vi "WaitForConnect.vi"(8 "error in (no error)":errorcluster, 11 "ServiceManager-Comms in":refnum<class "ServiceManager-Comms.lvclass">) -> (0 "error out":errorcluster, 3 "ServiceManager-Comms out":refnum<class "ServiceManager-Comms.lvclass">)   [LabVIEW 2020, in "ServiceManager.lvlib" / "ServiceManager-Comms.lvclass"]
uses:
  ServiceManager-Comms.lvclass
  C:/Program Files (x86)/National Instruments/LabVIEW 2020/vi.lib/ActorFramework/Actor/Actor.lvclass
  ServiceManager-Comms.lvclass/ServiceManager-Comms.ctl
  ServiceManager-Comms Messages/WaitForCommand Msg/WaitForCommand Msg.lvclass
  C:/Program Files (x86)/National Instruments/LabVIEW 2020/vi.lib/ActorFramework/Message/Message.lvclass
  ServiceManager-Comms Messages/WaitForConnect Msg/WaitForConnect Msg.lvclass
  <vilib>/ActorFramework/Actor/Actor.lvclass/Actor.ctl
  <vilib>/ActorFramework/Message Enqueuer/Message Enqueuer.lvclass/Message Enqueuer.ctl
  <vilib>/ActorFramework/Message Enqueuer/Init from Existing Queue.vi
  <vilib>/ActorFramework/Message Enqueuer/Message Enqueuer.lvclass
  <vilib>/ActorFramework/Actor/Actor.lvclass
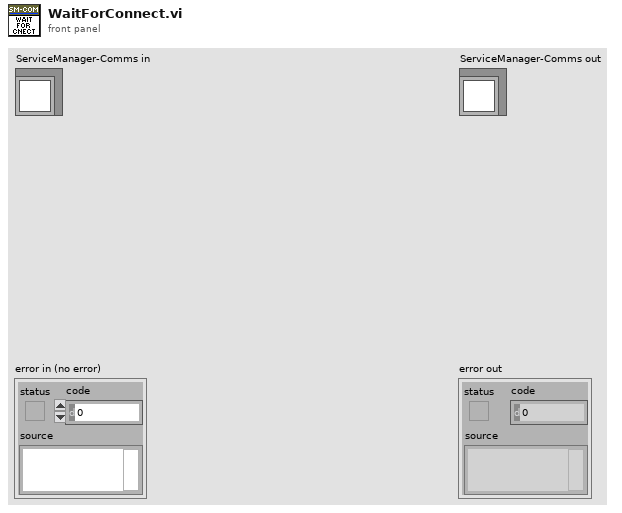
[diagram p1: front panel]
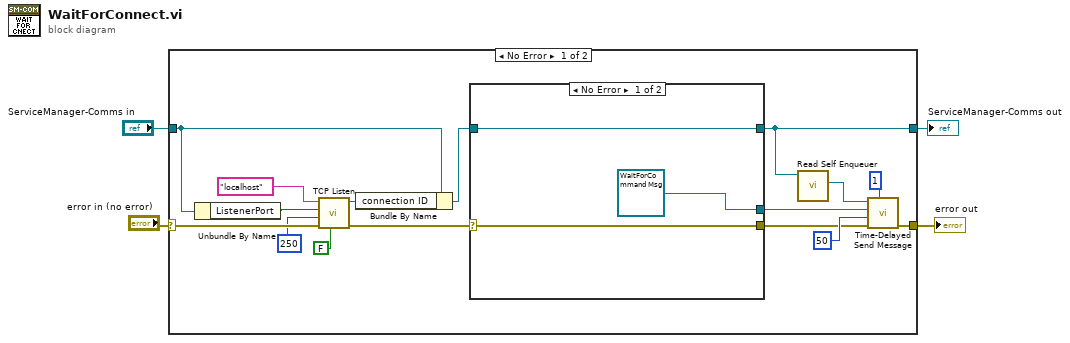
[diagram p0: block diagram]
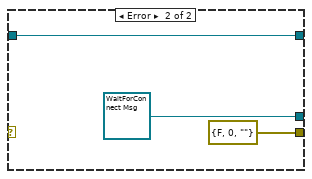
[diagram p2: hidden frame]
diagram:
  n1 = case shown="No Error" "error in (no error)" {
    selector: "error in (no error)" -> [w19 w28]
    tunnel: [w10 w28] -> w3
    tunnel: [w11 w27] -> w1
    tunnel: "ServiceManager-Comms in" -> [w16 w27]
    frame No Error {
      n2 = Unbundle By Name(w16) -> ("ListenerPort"=w18:u16)
      n3 = call <vilib>:"TCP Listen.vi"("resolve remote address (T)"=FALSE, "error in (no error)"=w19, "timeout ms (wait forever: -1)"=250, "port"=w18, "service name"="localhost") -> ("error out"=w13:errorcluster, "connection ID"=w15:refnum<k5>)  [unwired: 2 in, 3 out]
      n4 = Bundle By Name(cluster=w16, "connection ID"=w15) -> (w12:refnum<class "ServiceManager-Comms.lvclass">)
      n5 = case shown="No Error" w13 {
        selector: w13 -> [w22 _]
        tunnel: [w23 w26] -> w11
        tunnel: [w22 errorcluster {"status"=FALSE, "code"=0, "source"=""} ("error IO")] -> w6
        tunnel: w12 -> [w23 w26]
        tunnel: [refnum<class "WaitForCommand Msg.lvclass"> refnum ("ServiceManager.lvlib:WaitForCommand Msg.lvclass") refnum<class "WaitForConnect Msg.lvclass"> refnum ("ServiceManager.lvlib:WaitForConnect Msg.lvclass")] -> w8
        frame No Error {
        }
        frame Error {
        }
      }
      n6 = call <vilib>:"Read Self Enqueuer.vi"("Actor"=w11) -> ("Self Enqueuer"=w5:refnum<class "Message Enqueuer.lvclass">)  [unwired: 10 in]
      n7 = call <vilib>:"Time-Delayed Send Message.vi"("# Copies (0 = infinite repeat)"=u32 1, "error in (no error)"=w6, "Milliseconds To Wait"=50, "Message"=w8, "Message Enqueuer"=w5) -> ("error out"=w10:errorcluster)  [unwired: 5 in, 1 out]
    }
    frame Error {
    }
  }
  "error out" <- w3
  "ServiceManager-Comms out" <- w1
